vi "Test in Loop_0.vi"() -> ()   [LabVIEW 2020]
uses:
  99_Reference/LVMQTT-master/Controls/Connection_Return_Codes.ctl
  99_Reference/LVMQTT-master/Controls/User_Info.ctl
  99_Reference/LVMQTT-master/Controls/Connect_Flags.ctl
  99_Reference/LVMQTT-master/Controls/QoS.ctl
  99_Reference/LVMQTT-master/Controls/DUP_Flag.ctl
  99_Reference/LVMQTT-master/Controls/Retain_Flag.ctl
  <vilib>/NI/AMC/Read Termination Message.vi
  <vilib>/NI/AMC/Create Single Message.vi
  <vilib>/NI/AMC/Update Message Routing Info.vi
  <vilib>/NI/AMC/Globals.vi
  <vilib>/NI/AMC/Send Message.vi
  <vilib>/ErrorRing/Error Ring.xnode
  <vilib>/addons/JSON API/JSON Value/JSON Value.lvclass
  <vilib>/addons/JSON API/JSON Value/Get as JSON string (pretty).vi
  <vilib>/addons/JSON API/JSON Value/Set from JSON string.vi
  99_Reference/LVMQTT-master/MQTT_Functions.lvlib
  <vilib>/NI/AMC/AMC.lvlib
  <userlib>/_OpenG.lib/time/time.llb/openg_time.lvlib
  <vilib>/addons/JSON API/Get Polymorphic/JSON GetSet.lvlib
panel:
  in  "Read":bool
  out "ReadCMD_0":string="\u0000\u0001{\"ID\": \"fc6981fe-2619-4699-a965-530b28fed39b\", \"TO\": \"0050C500001E\", \"FROM\": \"C87F542F1180\", \"CMD\": 0, \"CONTENT\": [{\"HOSTNAME\": \"SI-AGT01\", \"MAC\": \"0050C500001E\", \"IP\": \"172.16.0.248\", \"CENTER_NAME\": \"C87F542F1180\", \"ADD_TOPIC\": \"topic/PC/0050C500001E\", \"REQ_ID\": \"88519866-1952-4B11-8249-306205650CEC\"}], \"STATUS\": true, \"ERRCODE\": \"\", \"ERRMSG\": \"\", \"TIMESTAMP\": 175887754"
  in  "CMD_0":bool
  in  "Test Connect":bool
  out "Connection Status":T1
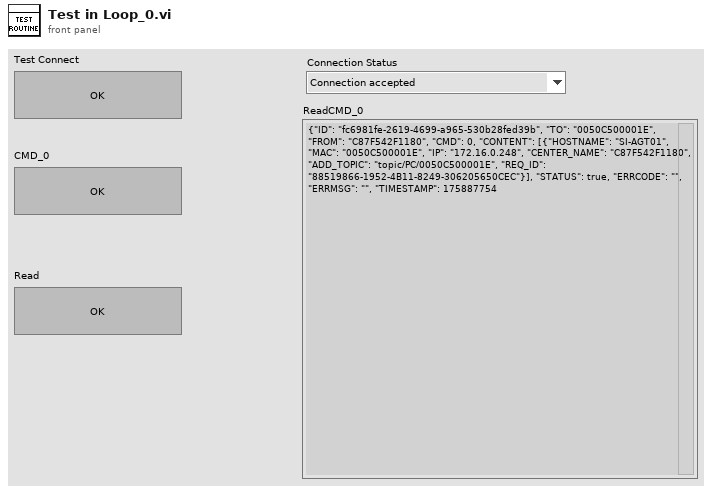
[diagram p1: front panel]
types:
  T1 = typedef "MQTT_Functions.lvlib/Connection_Return_Codes.ctl" = enum16{"Connection accepted", "Connection refused: unacceptable protocol version", "Connection refused: identifier rejected", "Connection refused: Server unavailable", "Connection refused: bad user name or password", "Connection refused: not authorized"}
  T2 = typedef "AMC.lvlib/Message Queue.ctl" = refnum<queue>
  T3 = typedef "MQTT_Functions.lvlib/QoS.ctl" = enum8{"At most once", "At least once", "Exactly once", "Reserved"}
  T4 = typedef "MQTT_Functions.lvlib/Retain_Flag.ctl" = bool
  T5 = typedef "MQTT_Functions.lvlib/DUP_Flag.ctl" = bool
  T6 = cluster{"Hostname":string, "Mac(From)":string, "IP":string, "ConnID":refnum<k5>}
  T7 = cluster{"QoS":T3, "DUP":T5, "Retain":T4, "Keep Alive (sec)":u16}
  T8 = typedef "MQTT_Functions.lvlib/Connect_Flags.ctl" = cluster{"user name":bool, "password":bool, "will retain":bool, "will flag":bool, "clean session":bool, "reserved":bool, "will QoS":T3}
  T9 = typedef "MQTT_Functions.lvlib/User_Info.ctl" = cluster{"User Name":string, "Password":string}
  T10 = cluster{"User Info":T9, "Client ID":string, "MQTT Broker":cluster{"address (IP)":string, "port":u16}, "Connection Status":T1, "Connect Flags":T8, "Connect Meta":cluster{"QoS":T3, "DUP":T5, "Retain":T4, "Keep Alive (sec)":u16}, "MainInfo":cluster{"Hostname":string, "Mac(From)":string, "IP":string, "ConnID":refnum<k5>}, "Topic":string, "tickCount":u32, "tickTarget":u32, "Message ID":u16}
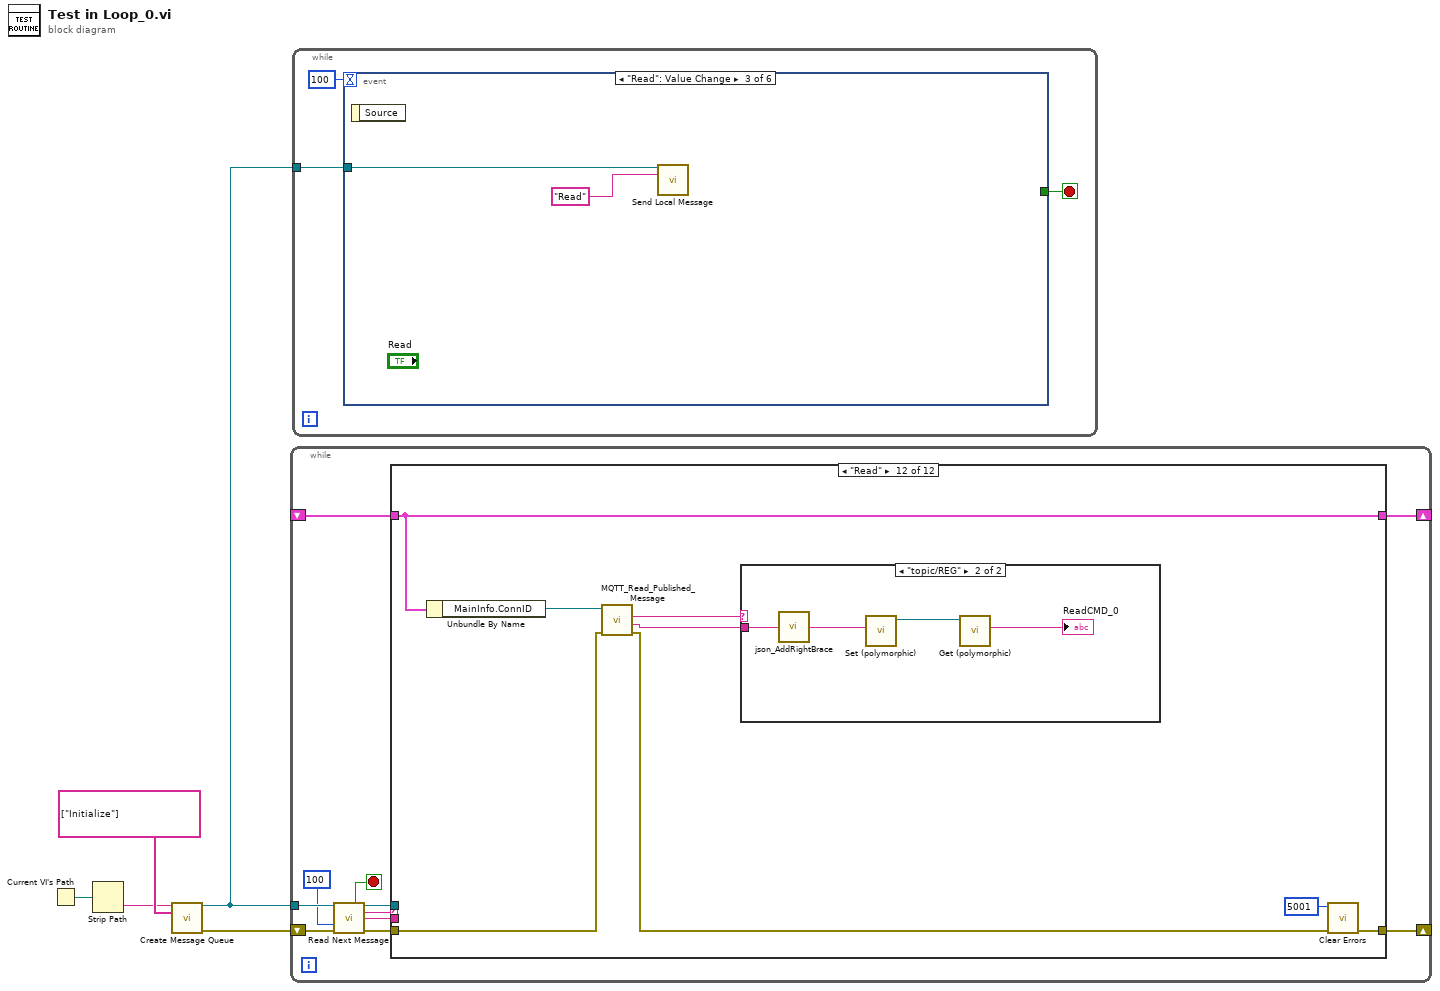
[diagram p0: block diagram]
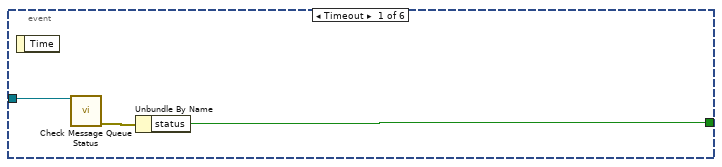
[diagram p2: hidden frame]
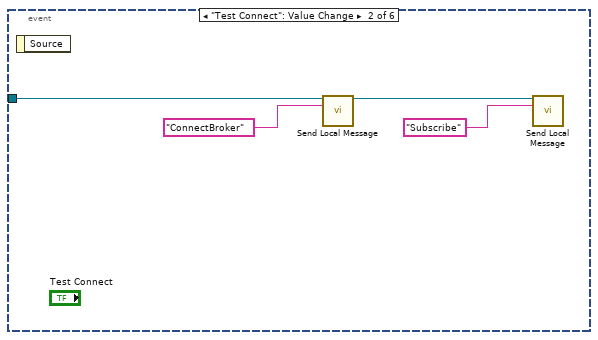
[diagram p3: hidden frame]
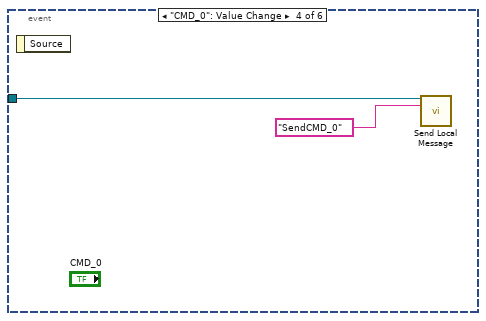
[diagram p4: hidden frame]
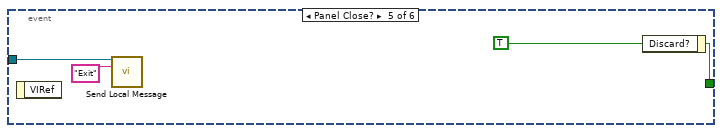
[diagram p5: hidden frame]
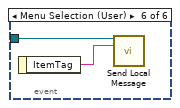
[diagram p6: hidden frame]
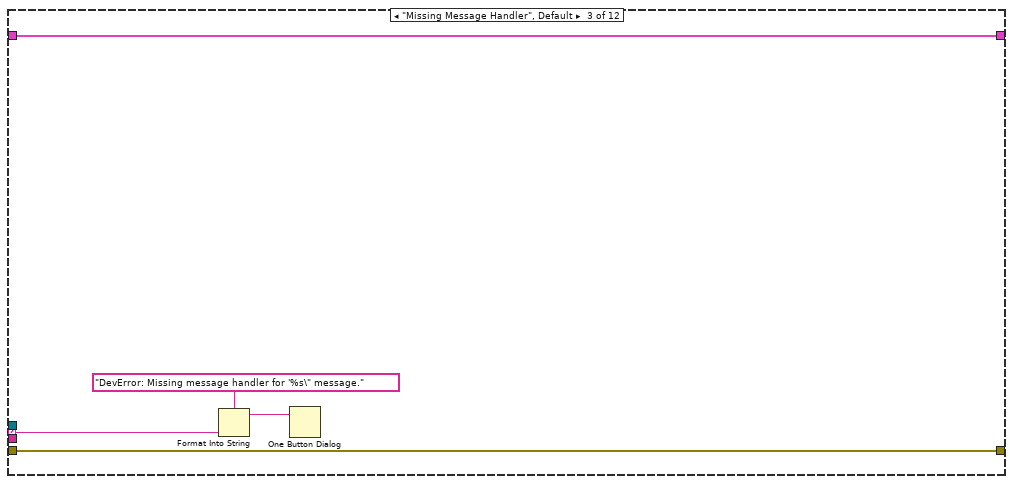
[diagram p9: hidden frame]
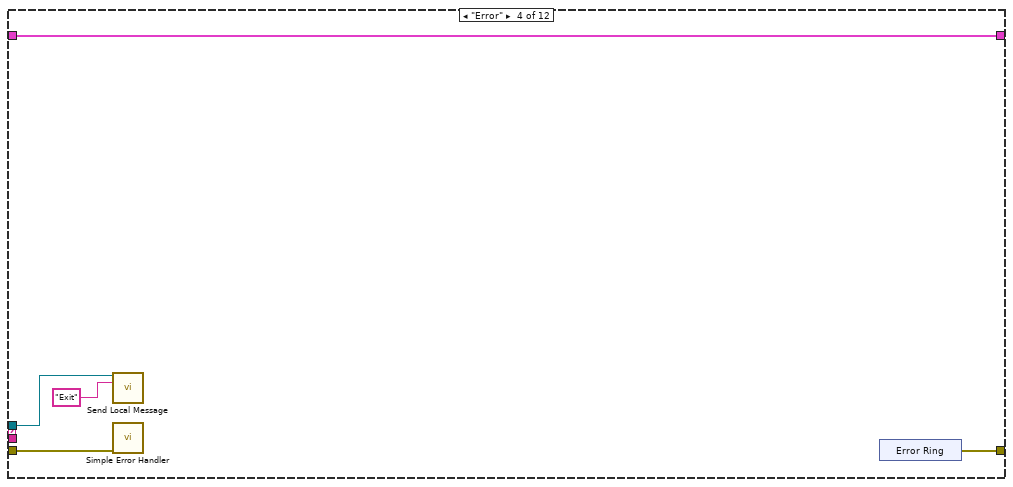
[diagram p10: hidden frame]
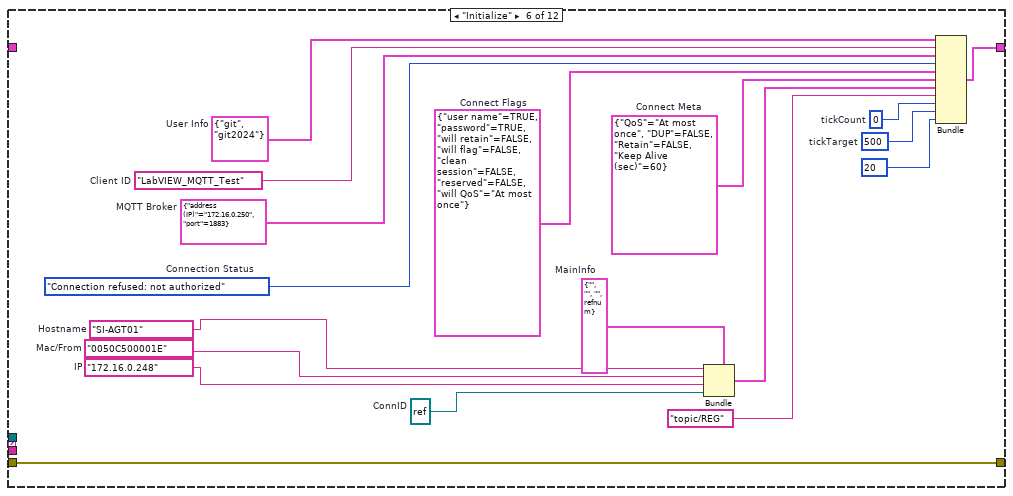
[diagram p12: hidden frame]
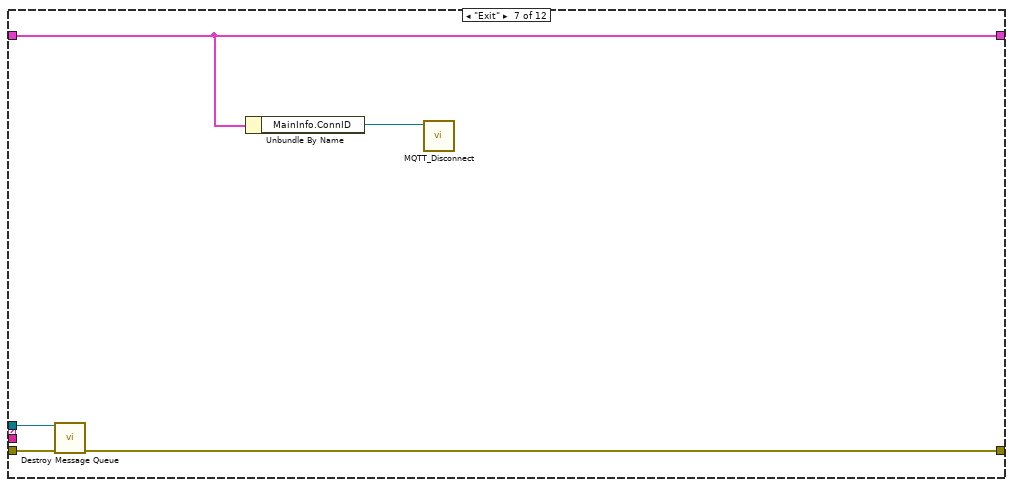
[diagram p13: hidden frame]
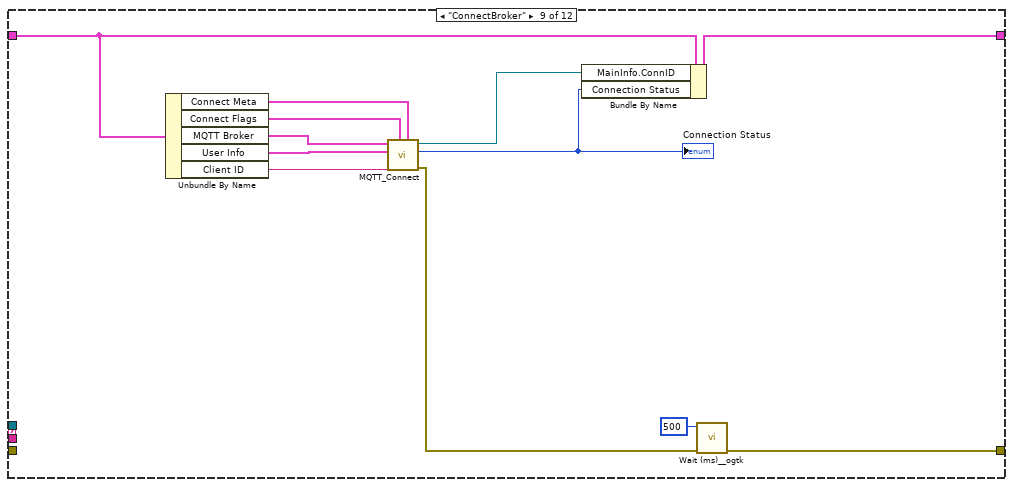
[diagram p15: hidden frame]
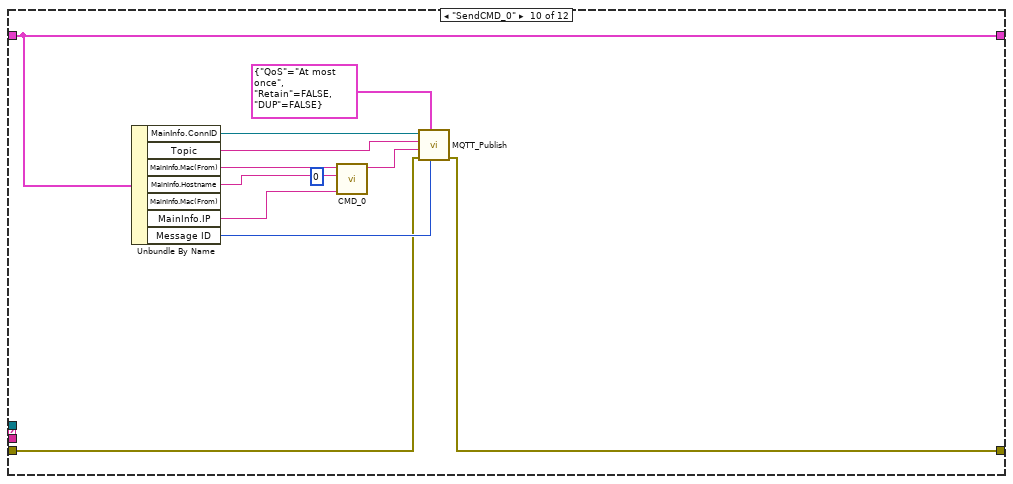
[diagram p16: hidden frame]
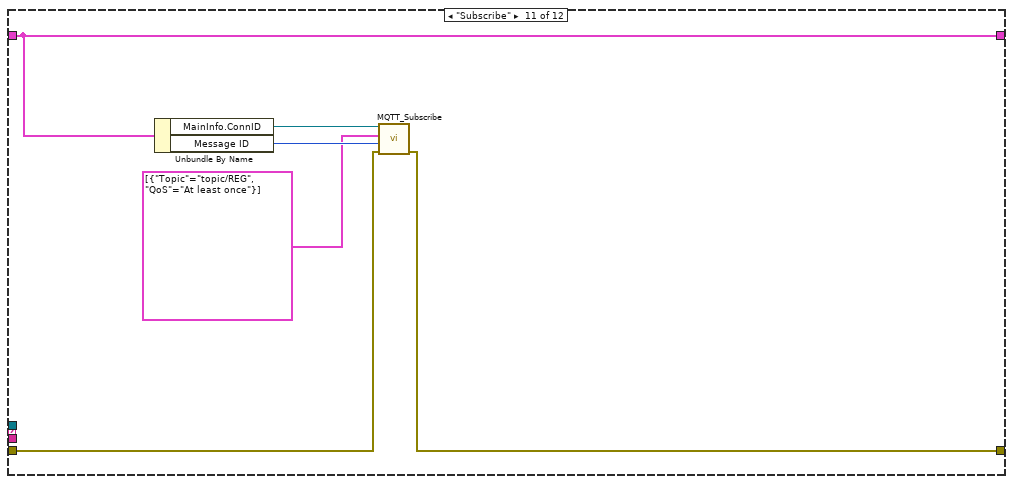
[diagram p17: hidden frame]
diagram:
  n1 = Current VI's Path() -> (path=w1:path)
  n2 = Strip Path(path=w1) -> (name=w4:string)  [unwired: 1 out]
  n3 = call <vilib>:"Create Message Queue.vi"("message queue name"=w4, "initial message names"=string[] ["Initialize"]) -> ("message queue out"=w3:T2, "error out"=w2:errorcluster)  [unwired: 12 in]
  n4 = while "Message Processor" {
    shift-left: w2 -> [w10]
    shift-right: [w14] -> _
    tunnel: w3 -> [w11]
    shift-left: _ -> [w16]
    shift-right: [w15] -> _
    stop <- w13 stop-if-true
    n5 = call <vilib>:"Read Next Message.vi"("message queue in"=w11, "timeout (1 ms)"=100 ("Timeout"), "error in"=w10) -> ("exit process?"=w13:bool, "message queue out"=w12:T2, "message name"=w8:string, "message value"=w7:string, "error out"=w9:errorcluster)  [unwired: 5 in, 3 out]
    n6 = case shown="\"Read\"" w8 {
      selector: w8 -> [_ _ w23 _ _ _ _ _ _ _ _ _]
      tunnel: [w18 w20 w25 w30 w33 w50 w53 w58 w65 w80 w88 w95] -> w15
      tunnel: w16 -> [w18 w20 w25 w30 w33 _ w53 w58 w70 w80 w88 w95]
      tunnel: w12 -> [_ _ _ w29 _ _ w55 _ _ _ _ _]
      tunnel: w9 -> [w17 w19 w24 w27 w32 w51 w56 w57 _ w71 w86 w89]
      tunnel: [w17 w19 w24 w26 w32 w51 w54 w57 w60 w78 w85 w91] -> w14
      tunnel: w7 -> [_ _ _ _ _ _ _ _ _ _ _ _]
      frame "---------- Framework Operations ----------" {
      }
      frame "", "Idle" {
      }
      frame "Missing Message Handler", Default {
        n7 = Format Into String(format string="DevError: Missing message handler for '%s\" message." ("message"), w23) -> (resulting string=w21:string)  [unwired: 2 in, 1 out]
        n8 = One Button Dialog(message=w21) -> ()  [unwired: 2 out]
      }
      frame "Error" {
        n9 = call <vilib>:"Send Local Message.vi"("message queue in"=w29, "message name"="Exit") -> ()  [unwired: 11 in, 3 out]
        n10 = call <vilib>:"Simple Error Handler.vi"("error in (no error)"=w27) -> ()  [unwired: 1 in, 8 out]
        n11 = xnode "Error Ring"() -> ("error out"=w26:errorcluster)
      }
      frame "---------- Generic Operations ----------" {
      }
      frame "Initialize" {
        w36 = "172.16.0.248"  # IP
        w35 = "0050C500001E"  # Mac/From
        w34 = "SI-AGT01"  # Hostname
        w38 = u32 500  # tickTarget
        w39 = u32 0  # tickCount
        w41 = T6 {"Hostname"="", "Mac(From)"="", "IP"="", "ConnID"=refnum}  # MainInfo
        w42 = refnum<k5> refnum  # ConnID
        w44 = T7 {"QoS"=enum."At most once", "DUP"=FALSE, "Retain"=FALSE, "Keep Alive (sec)"=60}  # Connect Meta
        w45 = T8 {"user name"=TRUE, "password"=TRUE, "will retain"=FALSE, "will flag"=FALSE, "clean session"=FALSE, "reserved"=FALSE, "will QoS"=enum."At most once"}  # Connect Flags
        w46 = Connection_Return_Codes."Connection refused: not authorized"  # Connection Status
        w47 = cluster{"address (IP)":string, "port":u16} {"address (IP)"="172.16.0.250", "port"=1883}  # MQTT Broker
        w48 = "LabVIEW_MQTT_Test"  # Client ID
        w49 = T9 {"User Name"="git", "Password"="git2024"}  # User Info
        n12 = Bundle(cluster=w41, "Hostname"=w34, "Mac(From)"=w35, "IP"=w36, "ConnID"=w42) -> (w43:T6)
        n13 = Bundle("User Info"=w49, "Client ID"=w48, "MQTT Broker"=w47, "Connection Status"=w46, "Connect Flags"=w45, "Connect Meta"=w44, "MainInfo"=w43, "Topic"="topic/REG", "tickCount"=w39, "tickTarget"=w38, "Message ID"=u16 20) -> (w50:T10)  [unwired: 1 in]
      }
      frame "Exit" {
        n14 = call <vilib>:"Destroy Message Queue.vi"("message queue in"=w55, "error in"=w56) -> ("error out"=w54:errorcluster)  [unwired: 11 in, 2 out]
        n15 = Unbundle By Name(w53) -> ("MainInfo.ConnID"=w52:refnum<k5>)
        n16 = call "MQTT_Disconnect.vi"("connection ID"=w52) -> ()  [unwired: 10 in, 1 out]
      }
      frame "---------- Application Operations ----------" {
        # "Dummy case to add a seperator in the Case Structure menu"
      }
      frame "ConnectBroker" {
        n17 = Unbundle By Name(w70) -> ("Connect Meta"=w63:T7, "Connect Flags"=w62:T8, "MQTT Broker"=w69:cluster{"address (IP)":string, "port":u16}, "User Info"=w68:T9, "Client ID"=w67:string)
        n18 = call "MQTT_Connect.vi"("Connect Meta"=w63, "Client ID"=w67, "Connect Flags"=w62, "User Info"=w68, "MQTT Broker"=w69) -> ("error out"=w66:errorcluster, "Connection Status"=w64:T1, "connection ID out"=w61:refnum<k5>)  [unwired: 4 in]
        "Connection Status" <- w64
        n19 = Bundle By Name(cluster=w70, "MainInfo.ConnID"=w61, "Connection Status"=w64) -> (w65:T10)
        n20 = call <userlib>:"Wait (ms)__ogtk.vi"("error in (no error)"=w66, "milliseconds to wait"=u32 500) -> ("error out"=w60:errorcluster)  [unwired: 8 in, 1 out]
      }
      frame "SendCMD_0" {
        n21 = Unbundle By Name(w80) -> ("MainInfo.ConnID"=w82:refnum<k5>, "Topic"=w79:string, "MainInfo.Mac(From)"=w76:string, "MainInfo.Hostname"=w75:string, "MainInfo.IP"=w74:string, "Message ID"=w73:u16)  [unwired: 1 out]
        n22 = call "CMD_0.vi"("CMD"=u32 0, "IP"=w74, "HOSTNAME"=w75, "MAC"=w76) -> ("JSON String"=w81:string)  [unwired: 7 in]
        n23 = call "MQTT_Publish.vi"("Message ID"=w73, "Publish Meta"=cluster{"QoS":T3, "Retain":T4, "DUP":T5} {"QoS"=enum."At most once", "Retain"=FALSE, "DUP"=FALSE}, "error in (no error)"=w71, "Message to be published"=w81, "Topic"=w79, "connection ID"=w82) -> ("error out"=w78:errorcluster)  [unwired: 4 in, 1 out]
      }
      frame "Subscribe" {
        n24 = Unbundle By Name(w88) -> ("MainInfo.ConnID"=w87:refnum<k5>, "Message ID"=w84:u16)
        n25 = call "MQTT_Subscribe.vi"("error in (no error)"=w86, "Message ID"=w84, "Subscription Info Array"=cluster{"Topic":string, "QoS":T3}[] [{"Topic"="topic/REG", "QoS"=enum."At least once"}], "connection ID"=w87) -> ("error out"=w85:errorcluster)  [unwired: 6 in, 1 out]
      }
      frame "Read" {
        n26 = Unbundle By Name(w95) -> ("MainInfo.ConnID"=w96:refnum<k5>)
        n27 = call "MQTT_Read_Published_Message.vi"("error in (no error)"=w89, "connection ID"=w96) -> ("error out"=w93:errorcluster, "Message"=w92:string, "Topic Name"=w94:string)  [unwired: 4 in, 3 out]
        n28 = case shown="\"topic/REG\"" w94 {
          tunnel: w92 -> [_ w98]
          frame "False", Default {
          }
          frame "topic/REG" {
            n29 = call "json_AddRightBrace.vi"("ReadCMD_0"=w98) -> ("+}"=w97:string)
            n30 = call-poly <vilib>:"Set (polymorphic).vi"("JSON stream"=w97) -> ("JSON Value out"=w100:refnum<class "JSON Value.lvclass">)  [unwired: 8 in, 2 out]
            n31 = call-poly <vilib>:"Get (polymorphic).vi"("JSON Value in"=w100) -> ("<JSON>"=→"ReadCMD_0":string)  [unwired: 9 in, 1 out]
          }
        }
        n32 = call <vilib>:"Clear Errors.vi"("error in (no error)"=w93, "specific error code to clear (0: all)"=5001) -> ("error out"=w91:errorcluster)  [unwired: 4 in, 1 out]
      }
    }
  }
  n33 = while "Message Generator - User Interface Event Handler" {
    tunnel: w3 -> [w101]
    stop <- w102 stop-if-true
    n34 = event shown="[2] \"Read\": Value Change" {
      selector: _ -> [_ _ _ _ _ _]
      dyn-events: _ -> [_ _ _ _ _ _]
      timeout: 100 ("Event Structure Timeout (ms)") -> [_ _ _ _ _ _]
      tunnel: [w104 _ _ _ w117 _] -> w102
      tunnel: w101 -> [w105 w110 w112 w114 w115 w118]
      event Timeout {
        n35 = event-data() -> ()  [unwired: 2 out]
        n36 = call <vilib>:"Check Message Queue Status.vi"("message queue in"=w105) -> ("error out"=w106:errorcluster)  [unwired: 10 in, 4 out]
        n37 = Unbundle By Name(w106) -> ("status"=w104:bool)
      }
      event "Test Connect": Value Change {
        n38 = event-data() -> ()  [unwired: 2 out]
        n39 = call <vilib>:"Send Local Message.vi"("message queue in"=w110, "message name"="ConnectBroker") -> ("message queue out"=w107:T2)  [unwired: 11 in, 2 out]
        n40 = call <vilib>:"Send Local Message.vi"("message queue in"=w107, "message name"="Subscribe") -> ()  [unwired: 11 in, 3 out]
      }
      event "Read": Value Change {
        n41 = event-data() -> ()  [unwired: 2 out]
        n42 = call <vilib>:"Send Local Message.vi"("message queue in"=w112, "message name"="Read") -> ()  [unwired: 11 in, 3 out]
      }
      event "CMD_0": Value Change {
        n43 = event-data() -> ()  [unwired: 2 out]
        n44 = call <vilib>:"Send Local Message.vi"("message queue in"=w114, "message name"="SendCMD_0") -> ()  [unwired: 11 in, 3 out]
      }
      event Panel Close? {
        w117 = TRUE ("Discard?")
        n45 = event-data() -> ()  [unwired: 2 out]
        n46 = call <vilib>:"Send Local Message.vi"("message queue in"=w115, "message name"="Exit") -> ()  [unwired: 11 in, 3 out]
        n47 = event-data("Discard?"=w117) -> ()  [unwired: 1 in, 1 out]
      }
      event Menu Selection (User) {
        n48 = event-data() -> ("ItemTag"=w119:string)  [unwired: 1 out]
        n49 = call <vilib>:"Send Local Message.vi"("message queue in"=w118, "message name"=w119) -> ()  [unwired: 11 in, 3 out]
      }
    }
  }
